vi "UpdateLinkCameraStatus.vi"(8 "error in (no error)":errorcluster, 10 "LinkCameraStatus":T1=enum."Connected", 11 "CameraTestingUI in":refnum<class "CameraTestingUI.lvclass">) -> (0 "error out":errorcluster, 3 "CameraTestingUI out":refnum<class "CameraTestingUI.lvclass">)   [LabVIEW 2020, in "CameraTestingUI.lvlib" / "CameraTestingUI.lvclass"]
uses:
  CameraTestingUI.lvclass
  ICameraTestingUI/ICameraTestingUI/TypeDef/LinkCameraStatus.ctl
  CameraTestingUI.lvclass/CameraTestingUI.ctl
  ICameraTestingUI/ICameraTestingUI/ICameraTestingUI.lvclass
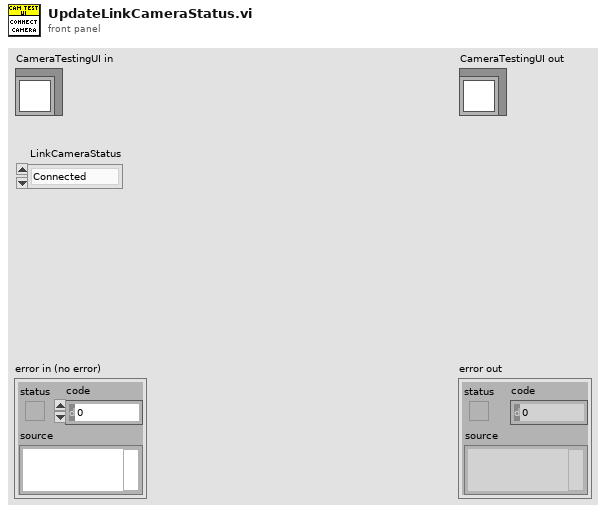
[diagram p1: front panel]
types:
  T1 = typedef "ICameraTestingUI.lvlib/ICameraTestingUI.lvclass/LinkCameraStatus.ctl" = enum8{"Disconnected", "Connected", "Error"}
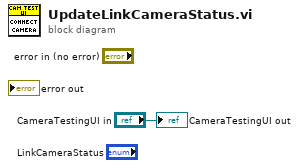
[diagram p0: block diagram]
diagram:
  "CameraTestingUI out" <- "CameraTestingUI in"
